vi "Caraya CLI.vi"() -> ()   [LabVIEW 2013]
uses:
  Caraya.lvlib
panel:
  out "quit":bool
  out "error out":errorcluster
  out "source folder":path
  out "report filename":string
  out "Application:Command Line Arguments":string[](array[string])
  out "recursive":bool
  out "verbose":bool
  out "Interactive":bool
  out "output path":path
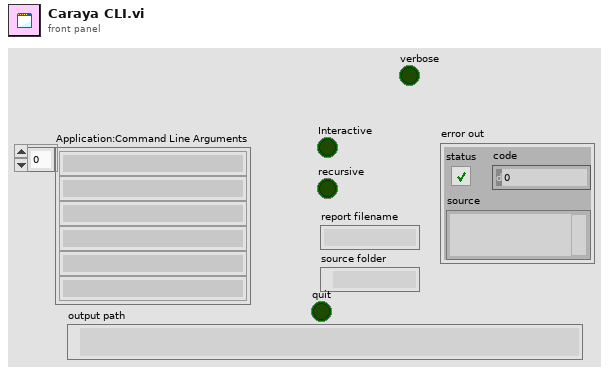
[diagram p1: front panel]
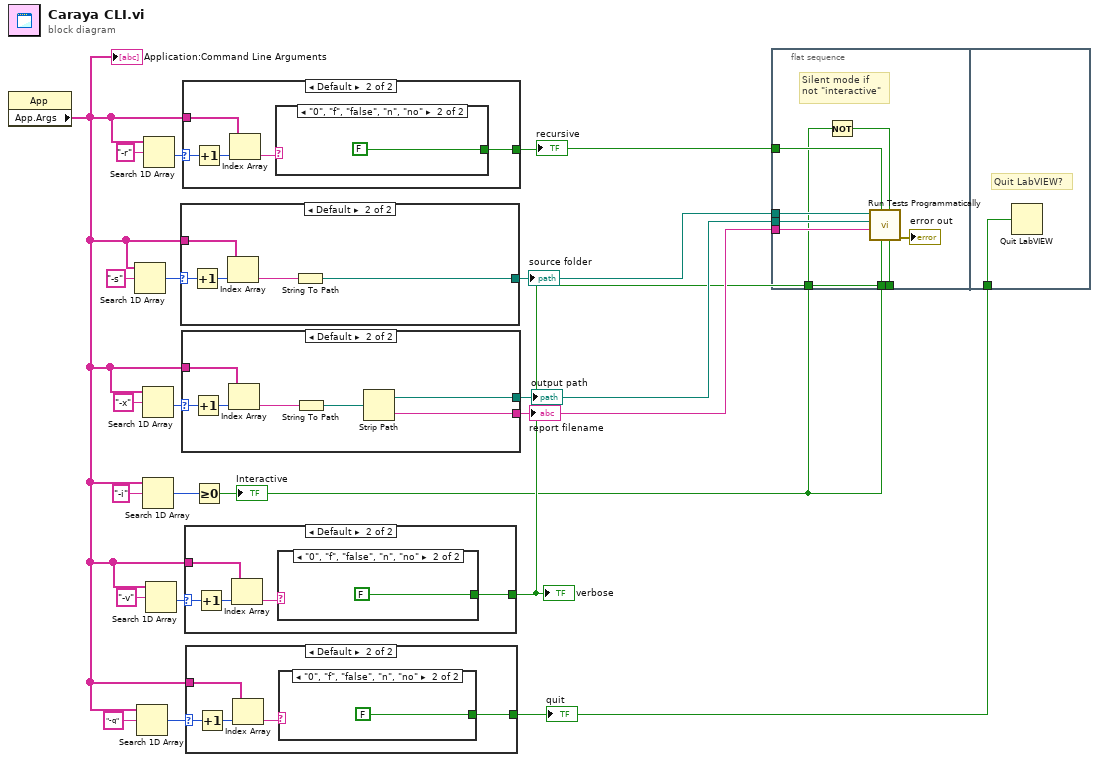
[diagram p0: block diagram]
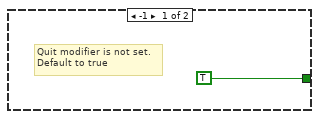
[diagram p2: hidden frame]
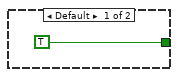
[diagram p3: hidden frame]
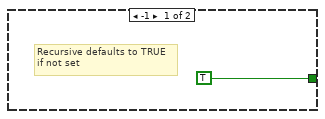
[diagram p6: hidden frame]
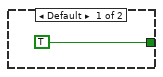
[diagram p7: hidden frame]
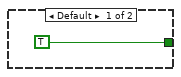
[diagram p9: hidden frame]
diagram:
  n1 = property class="App"() -> ("App.Args"=w3:string[])  [unwired: 2 in, 2 out]
  "Application:Command Line Arguments" <- w3
  n2 = Search 1D Array(1D array=w3, element="-s") -> (index of element=w11:i32)  [unwired: 1 in]
  n3 = Search 1D Array(1D array=w3, element="-q") -> (index of element=w2:i32)  [unwired: 1 in]
  n4 = Search 1D Array(1D array=w3, element="-x") -> (index of element=w13:i32)  [unwired: 1 in]
  n5 = Search 1D Array(1D array=w3, element="-i") -> (index of element=w19:i32)  [unwired: 1 in]
  n6 = Search 1D Array(1D array=w3, element="-r") -> (index of element=w16:i32)  [unwired: 1 in]
  n7 = Search 1D Array(1D array=w3, element="-v") -> (index of element=w17:i32)  [unwired: 1 in]
  n8 = case shown="Default" w11 {
    selector: w11 -> [_ w24]
    tunnel: w3 -> [_ w23]
    tunnel: [_ w21] -> w10
    frame -1 {
    }
    frame Default {
      n9 = Increment(x=w24) -> (x+1=w25:i32)
      n10 = Index Array(array=w23, index=w25) -> (element=w22:string)
      n11 = String To Path(string=w22) -> (path=w21:path)
    }
  }
  "source folder" <- w10
  n12 = case shown="Default" w13 {
    selector: w13 -> [_ w31]
    tunnel: w3 -> [_ w30]
    tunnel: [_ w27] -> w9
    tunnel: [_ w26] -> w8
    frame -1 {
    }
    frame Default {
      n13 = Increment(x=w31) -> (x+1=w32:i32)
      n14 = Index Array(array=w30, index=w32) -> (element=w29:string)
      n15 = String To Path(string=w29) -> (path=w28:path)
      n16 = Strip Path(path=w28) -> (stripped path=w27:path, name=w26:string)
    }
  }
  "output path" <- w9
  "report filename" <- w8
  n17 = case shown="Default" w16 {
    selector: w16 -> [_ w35]
    tunnel: [TRUE w36] -> w7
    tunnel: w3 -> [_ w34]
    frame -1 {
      # "Recursive defaults to TRUE\nif not set"
    }
    frame Default {
      n18 = Increment(x=w35) -> (x+1=w38:i32)
      n19 = Index Array(array=w34, index=w38) -> (element=w37:string)
      n20 = case shown="\"0\", \"f\", \"false\", \"n\", \"no\"" w37 {
        tunnel: [TRUE FALSE] -> w36
        frame Default {
        }
        frame "0", "f", "false", "n", "no" {
        }
      }
    }
  }
  "recursive" <- w7
  n21 = case shown="Default" w17 {
    selector: w17 -> [_ w42]
    tunnel: [_ w43] -> w6
    tunnel: w3 -> [_ w41]
    frame -1 {
      # "Verosity defaults to False\nif not set"
    }
    frame Default {
      n22 = Increment(x=w42) -> (x+1=w45:i32)
      n23 = Index Array(array=w41, index=w45) -> (element=w44:string)
      n24 = case shown="\"0\", \"f\", \"false\", \"n\", \"no\"" w44 {
        tunnel: [TRUE FALSE] -> w43
        frame Default {
        }
        frame "0", "f", "false", "n", "no" {
        }
      }
    }
  }
  "verbose" <- w6
  n25 = case shown="Default" w2 {
    selector: w2 -> [_ w50]
    tunnel: [TRUE w51] -> w1
    tunnel: w3 -> [_ w49]
    frame -1 {
      # "Quit modifier is not set.\nDefault to true"
    }
    frame Default {
      n26 = Increment(x=w50) -> (x+1=w53:i32)
      n27 = Index Array(array=w49, index=w53) -> (element=w52:string)
      n28 = case shown="\"0\", \"f\", \"false\", \"n\", \"no\"" w52 {
        tunnel: [TRUE FALSE] -> w51
        frame Default {
        }
        frame "0", "f", "false", "n", "no" {
        }
      }
    }
  }
  "quit" <- w1
  n29 = Greater Or Equal To 0?(x=w19) -> (x >= 0?=w5:bool)
  "Interactive" <- w5
  n30 = flat-sequence {
    tunnel: w10 -> [w64]
    tunnel: w9 -> [w63]
    tunnel: w8 -> [w62]
    tunnel: w7 -> [w61]
    tunnel: w5 -> [w60]
    tunnel: w6 -> [w59]
    tunnel: w5 -> [w58]
    tunnel: w1 -> [w65]
    frame #0 {
      # "Silent mode if\nnot \"interactive\""
      n31 = Not(x=w58) -> (.not. x?=w57:bool)
      n32 = call "Run Tests Programmatically.vi"("Verbose"=w59, "Silent"=w57, "Interactive"=w60, "Inspect Recursively"=w61, "Report name"=w62, "Output Folder"=w63, "Source Folder"=w64) -> ("error out"=→"error out":errorcluster)  [unwired: 3 in, 1 out]
    }
    frame #1 {
      # "Quit LabVIEW?"
      n33 = Quit LabVIEW(quit? (T)=w65) -> ()
    }
  }
